vi "ProfileXY.vi"() -> ()   [LabVIEW 2009]
panel:
  out "Threshold":cluster{"max":u32, "min":u32}
  out "RGB/Flase":bool
  out "x-max Pos":i32
  out "x-max":u32
  out "y-max Pos":i32
  out "y-max":u32
  in  "Coordinates":i32[](array[numeric])
  out "y-direction":u32[][](graph)
  out "x-direction":u32[][](graph)
  in  "stop":bool
  in  "plane":i32
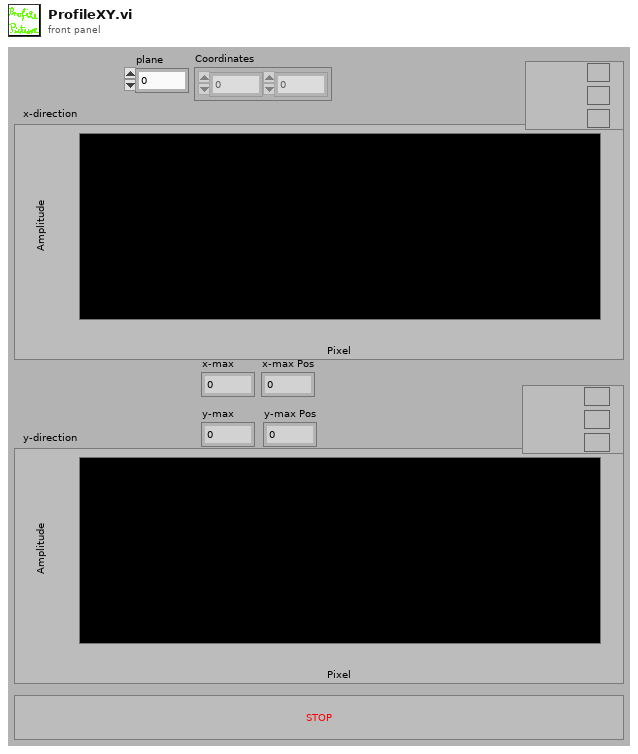
[diagram p1: front panel]
types:
  T1 = enum16{"Display", "change", "Get", "Set", "Set Ken"}
  T2 = enum16{"Get", "Set", "Change", "ini", "clear", "draw", "draw false"}
  T3 = cluster{"Name":string, "Color":u32, "Hair Style":u8, "Point Style":u8, "Name Visible":bool, "Trackable":bool, "Lock Style":u32, "Plot Number":u32, "Marker Index":i32, "Location":cluster{"X":dbl, "Y":dbl}}
  T4 = typedef "IMAQ Image.ctl" = refnum<image>
  T5 = typedef "FIFOSettings_BH.ctt" = cluster{"Measurement":cluster{"Binning (ms)":sgl, "External Trigger Condition":u16, "Stop Condition:":u16, "Stop Count":dbl, "Buffer Size (Photons)":u16, "No of Channels":u16, "Ext Latch Delay":i16}, "ADC":cluster{"Module":u16, "ADC Resolution":i32, "Dither Range":i16, "Count Increment":i16, "Macro Time Clock":i16}, "SYNC":cluster{"SYNC ZC Level (mV)":sgl, "SYNC Freq Divider":i16, "SYNC Holdoff (ns)":sgl, "SYNC Threshold (mV)":sgl}, "TAC":cluster{"TAC Range (ns)":sgl, "TAC Gain":i16, "TAC Offset (%)":sgl, "TAC Limit Low (%)":sgl, "TAC Limit High (%)":sgl}, "CFD":cluster{"CFD Limit Low (mV)":sgl, "CFD Limit High (mV)":sgl, "CFD ZC Level (mV)":sgl, "CFD Holdoff (ns)":sgl}}
  T6 = cluster{"Name":string, "Color":u32, "Hair Style":u8, "Point Style":u8, "Name Visible":bool, "Trackable":bool, "Lock Style":u32, "Plot Number":u32, "Marker Index":i32, "Location":cluster{"X":dbl, "Y":dbl}}[]
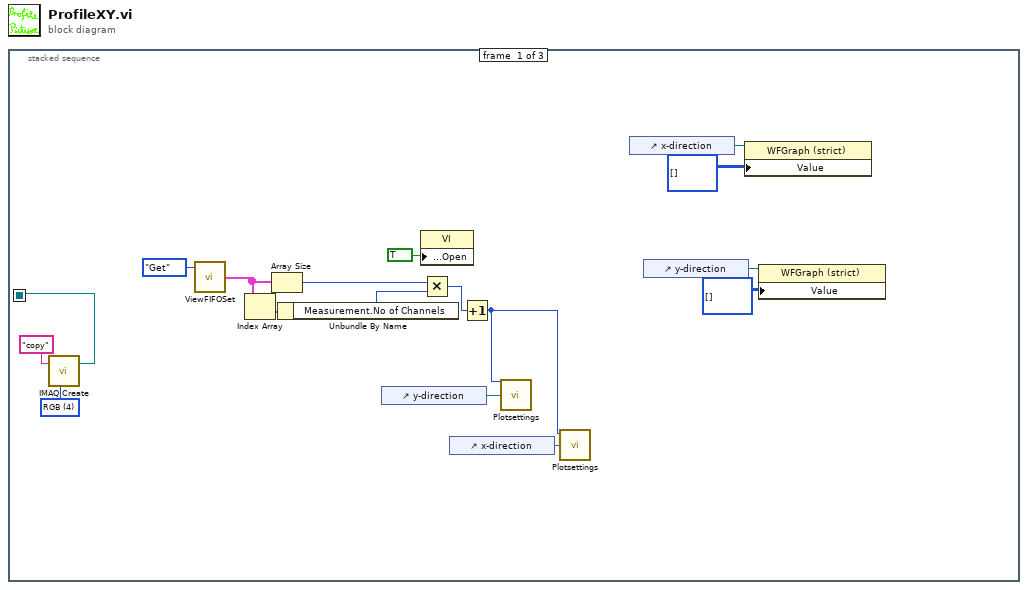
[diagram p0: block diagram]
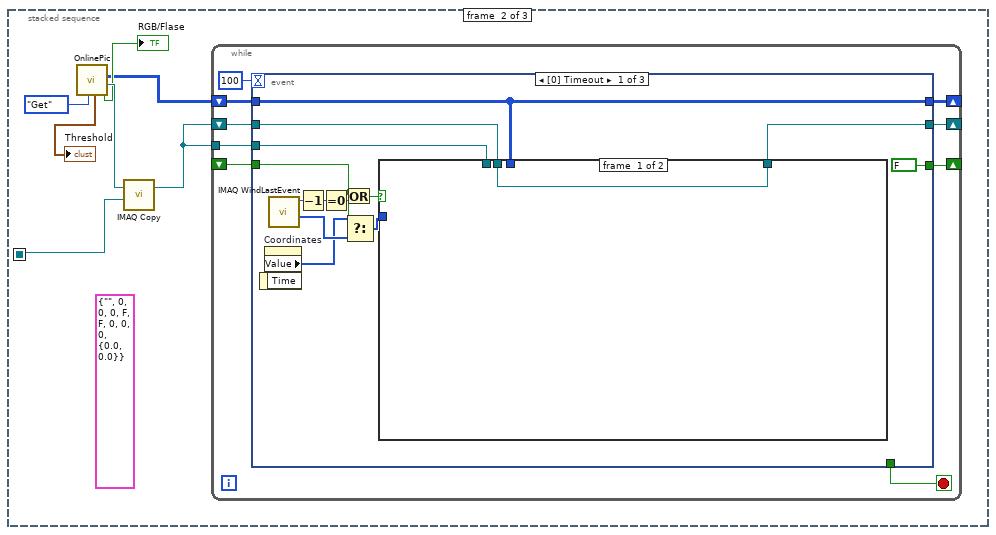
[diagram p2: hidden frame]
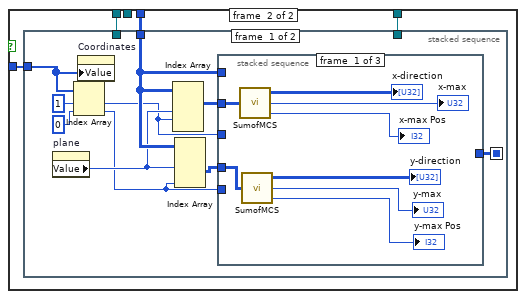
[diagram p3: hidden frame]
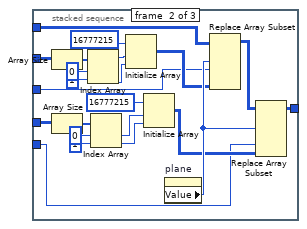
[diagram p4: hidden frame]
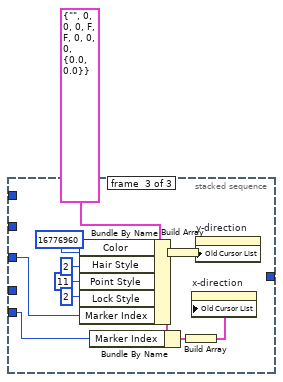
[diagram p5: hidden frame]
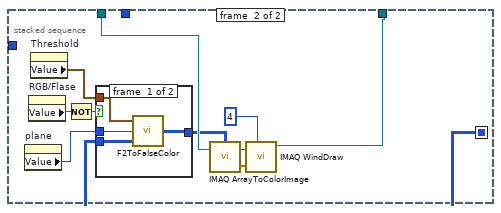
[diagram p6: hidden frame]
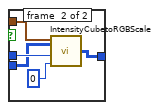
[diagram p7: hidden frame]
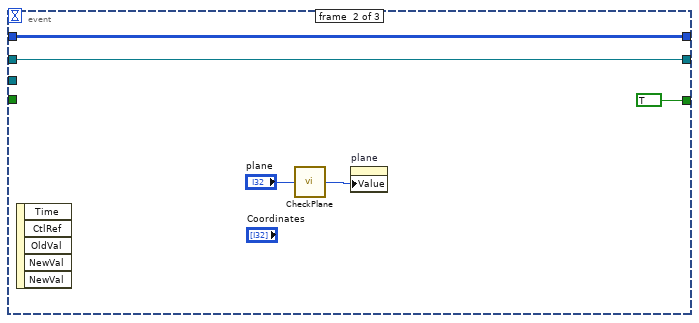
[diagram p8: hidden frame]
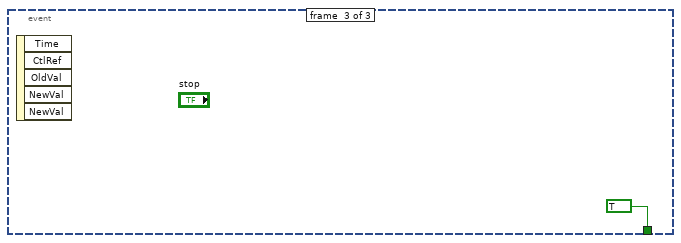
[diagram p9: hidden frame]
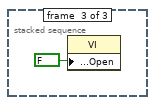
[diagram p10: hidden frame]
diagram:
  n1 = stacked-sequence {
    seq-local: [w16 _ _] -> [_ w22 _]
    frame #0 {
      w15 = u32 4 items=["8 bits", "16 bits", "Float", "Complex", "RGB", "HSL"] ("Image Type")
      n2 = call "IMAQ Create"("Image Name"="copy", "Image Type"=w15) -> ("New Image"=w16:T4)  [unwired: 3 in, 1 out]
      n3 = call "ViewFIFOSet.vi"("Enum"=T1."Get") -> ("FIFO Settings (Array)"=w4:T5[])  [unwired: 1 in]
      n4 = Index Array(array=w4) -> (element=w5:T5)  [unwired: 1 in]
      n5 = Array Size(array=w4) -> (size(s)=w2:i32)
      n6 = Unbundle By Name(w5) -> ("Measurement.No of Channels"=w3:u16)
      n7 = control-ref of="y-direction"() -> (w13:refnum<vi>)
      n8 = property class="VI"("Front Panel Window:Open"=TRUE) -> ()  [unwired: 2 in, 2 out]
      n9 = Multiply(x=w2, y=w3) -> (x*y=w1:i32)
      n10 = control-ref of="x-direction"() -> (w12:refnum<vi>)
      n11 = Increment(x=w1) -> (x+1=w10:i32)
      n12 = call "Plotsettings.vi"("Decays 2"=w13, "No of Channels"=w10) -> ()  [unwired: 4 in]
      n13 = call "Plotsettings.vi"("Decays 2"=w12, "No of Channels"=w10) -> ()  [unwired: 4 in]
      n14 = control-ref of="x-direction"() -> (w9:refnum<vi>)
      n15 = control-ref of="y-direction"() -> (w8:refnum<vi>)
      n16 = property class="WFGraph (strict)"(reference=w9, "Value"=u32[][] []) -> ()  [unwired: 1 in, 2 out]
      n17 = property class="WFGraph (strict)"(reference=w8, "Value"=u32[][] []) -> ()  [unwired: 1 in, 2 out]
    }
    frame #1 {
      (unwired) T3 {"Name"="", "Color"=0, "Hair Style"=0, "Point Style"=0, "Name Visible"=FALSE, "Trackable"=FALSE, "Lock Style"=0, "Plot Number"=0, "Marker Index"=0, "Location"={"X"=0.0, "Y"=0.0}}
      n18 = call "OnlinePic.vi"("action"=T2."Get" ("Enum")) -> ("Image Out (duplicate)"=w23:T4, "Sum of Photons"=w19:u32[][][][], "RGB/False out"=→"RGB/Flase":bool, "Threshold (max) OUT"=→"Threshold":cluster{"max":u32, "min":u32})  [unwired: 6 in, 1 out]
      n19 = call "IMAQ Copy"("Image Dst"=w22, "Image Src"=w23) -> ("Image Dst Out"=w20:T4)  [unwired: 4 in, 1 out]
      n20 = while {
        shift-right: [w32] -> _
        shift-left: w19 -> [w31]
        tunnel: w20 -> [w29]
        shift-right: [w27] -> _
        shift-left: w20 -> [w28]
        shift-right: [w26] -> _
        shift-left: _ -> [w25]
        stop <- w33 stop-if-true
        n21 = event shown="[0] Timeout" {
          selector: _ -> [_ _ _]
          dyn-events: _ -> [_ _ _]
          timeout: 100 -> [_ _ _]
          tunnel: [_ _ TRUE] -> w33
          tunnel: [w44 w126 _] -> w32
          tunnel: w31 -> [w44 w126 _]
          tunnel: w29 -> [w43 _ _]
          tunnel: w28 -> [w42 w127 _]
          tunnel: [w41 w127 _] -> w27
          tunnel: [FALSE TRUE _] -> w26
          tunnel: w25 -> [w36 _ _]
          event #0 {
            n22 = event-data() -> ()  [unwired: 1 in, 1 out]
            n23 = property on="Coordinates" class="Array (strict)"() -> ("Value"=w34:i32[])  [unwired: 2 in, 2 out]
            n24 = call "IMAQ WindLastEvent"() -> ("Coordinates"=w35:i32[], "Event"=w46:i32)  [unwired: 6 in, 4 out]
            n25 = Decrement(x=w46) -> (x-1=w45:i32)
            n26 = Equal To 0?(x=w45) -> (x = 0?=w40:bool)
            n27 = Or(x=w36, y=w40) -> (x .or. y?=w39:bool)
            n28 = Select(t=w34, s=w36, f=w35) -> (s? t:f=w37:i32[])
            n29 = case shown="True" w39 {
              tunnel: w37 -> [_ w51]
              tunnel: w44 -> [_ w50]
              tunnel: w43 -> [_ w49]
              tunnel: [w47 w48] -> w41
              tunnel: w42 -> [w47 _]
              frame #0 {
              }
              frame #1 {
                n30 = stacked-sequence {
                  seq-local: [w56 _] -> [_ w104]
                  tunnel: w51 -> [w52 _]
                  tunnel: w50 -> [w57 _]
                  tunnel: w49 -> [_ w111]
                  tunnel: [_ w107] -> w48
                  frame #0 {
                    n31 = property on="plane" class="DigNum (strict)"() -> ("Value"=w55:i32)  [unwired: 2 in, 2 out]
                    n32 = Index Array(array=w52, index #1=1 ("index"), index #2=0 ("index")) -> (element #1=w54:i32, element #2=w53:i32)
                    n33 = property on="Coordinates" class="Array (strict)"("Value"=w52) -> ()  [unwired: 2 in, 2 out]
                    n34 = Index Array(array=w57, index (dim 1)=w55, index (dim 2)=w54) -> (element=w58:u32[][])  [unwired: 2 in]
                    n35 = Index Array(array=w57, index (dim 1)=w55, index (dim 3)=w53) -> (element=w59:u32[][])  [unwired: 2 in]
                    n36 = stacked-sequence {
                      tunnel: w59 -> [w62 w86 _]
                      tunnel: w58 -> [w63 w87 _]
                      tunnel: w57 -> [_ w89 _]
                      tunnel: w54 -> [_ w71 w95]
                      tunnel: w53 -> [_ w70 w94]
                      tunnel: [_ w90 _] -> w56
                      frame #0 {
                        n37 = call "SumofMCS.vi"("Sum of Photons"=w63) -> ("MCS incl. sum"=→"x-direction":u32[][], "max value"=→"x-max":u32, "max index (indices)"=→"x-max Pos":i32)
                        n38 = call "SumofMCS.vi"("Sum of Photons"=w62) -> ("MCS incl. sum"=→"y-direction":u32[][], "max value"=→"y-max":u32, "max index (indices)"=→"y-max Pos":i32)
                      }
                      frame #1 {
                        n39 = Array Size(array=w87) -> (size(s)=w80:i32[])
                        n40 = Array Size(array=w86) -> (size(s)=w81:i32[])
                        n41 = Index Array(array=w80, index #1=0 ("index"), index #2=1 ("index")) -> (element #1=w73:i32, element #2=w72:i32)
                        n42 = Index Array(array=w81, index #1=0 ("index"), index #2=1 ("index")) -> (element #1=w75:i32, element #2=w74:i32)
                        n43 = Initialize Array(u32 16777215 ("element"), w73, w72) -> (w83:u32[][])
                        n44 = Initialize Array(u32 16777215 ("element"), w75, w74) -> (w82:u32[][])
                        n45 = property on="plane" class="DigNum (strict)"() -> ("Value"=w88:i32)  [unwired: 2 in, 2 out]
                        n46 = Replace Array Subset(array=w89, new element=w83, index (dim 1)=w88, index (dim 2)=w71) -> (w91:u32[][][][])  [unwired: 2 in]
                        n47 = Replace Array Subset(array=w91, new element=w82, index (dim 1)=w88, index (dim 3)=w70) -> (w90:u32[][][][])  [unwired: 2 in]
                      }
                      frame #2 {
                        n48 = Bundle By Name(cluster=T3 {"Name"="", "Color"=0, "Hair Style"=0, "Point Style"=0, "Name Visible"=FALSE, "Trackable"=FALSE, "Lock Style"=0, "Plot Number"=0, "Marker Index"=0, "Location"={"X"=0.0, "Y"=0.0}}, "Color"=u32 16776960 ("Cursor Color"), "Hair Style"=u8 2, "Point Style"=u8 11, "Lock Style"=u32 2, "Marker Index"=w95) -> (w102:T3)
                        n49 = Bundle By Name(cluster=w102, "Marker Index"=w94) -> (w93:T3)
                        n50 = Build Array(w102) -> (w100:T6)
                        n51 = Build Array(w93) -> (w92:T6)
                        n52 = property on="x-direction" class="WFGraph (strict)"("Old Cursor List"=w92) -> ()  [unwired: 2 in, 2 out]
                        n53 = property on="y-direction" class="WFGraph (strict)"("Old Cursor List"=w100) -> ()  [unwired: 2 in, 2 out]
                      }
                    }
                  }
                  frame #1 {
                    n54 = property on="plane" class="DigNum (strict)"() -> ("Value"=w103:i32)  [unwired: 2 in, 2 out]
                    n55 = property on="RGB/Flase" class="Boolean (strict)"() -> ("Value"=w113:bool)  [unwired: 2 in, 2 out]
                    n56 = property on="Threshold" class="Clust (strict)"() -> ("Value"=w112:cluster{"max":u32, "min":u32})  [unwired: 2 in, 2 out]
                    n57 = Not(x=w113) -> (.not. x?=w105:bool)
                    n58 = case shown="False" w105 {
                      tunnel: w112 -> [w117 w122]
                      tunnel: [w116 w121] -> w110
                      tunnel: w104 -> [w115 w119]
                      tunnel: w103 -> [w114 w120]
                      frame #0 {
                        n59 = call "F2ToFalseColor.vi"("Intensity"=w115, "Plane"=w114, "Threshold (max)"=w117) -> ("FalseColor"=w116:u32[][])
                      }
                      frame #1 {
                        n60 = call "IntensityCubetoRGBScale.vi"("Router"=u32 0, "Plane"=w120, "Trace"=w119, "threshold"=w122) -> ("RGB Scale"=w121:u32[][])
                      }
                    }
                    n61 = call "IMAQ ArrayToColorImage"("Image Pixels (U32)"=w110, "Image"=w111) -> ("Image Out"=w108:T4, "error out"=w109:errorcluster)  [unwired: 3 in]
                    n62 = call "IMAQ WindDraw"("Window Number (0...15)"=4, "error in (no error)"=w109, "Image"=w108) -> ("Image Out (duplicate)"=w107:T4)  [unwired: 7 in, 1 out]
                  }
                }
              }
            }
          }
          event #1 {
            n63 = event-data() -> ()  [unwired: 1 in, 5 out]
            n64 = call "CheckPlane.vi"("plane 2"="plane") -> ("plane"=w124:u32)
            n65 = property on="plane" class="Digital (strict)"("Value"=w124) -> ()  [unwired: 2 in, 2 out]
          }
          event #2 {
            n66 = event-data() -> ()  [unwired: 1 in, 5 out]
          }
        }
      }
    }
    frame #2 {
      n67 = property class="VI"("Front Panel Window:Open"=FALSE) -> ()  [unwired: 2 in, 2 out]
    }
  }
